vi "Replace Array Element (by ref) [U32].vi"(8 "Error In":errorcluster, 9 "Index":i32, 10 "New Element":u32, 11 "Array in":refnum<vi>) -> (0 "Error Out":errorcluster, 3 "Array out":refnum<vi>)   [LabVIEW 2021, in "Arrays.lvlib"]
uses:
  Arrays.lvlib
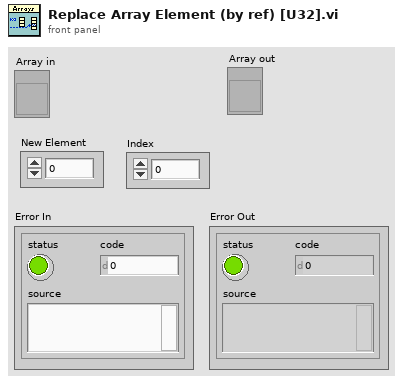
[diagram p1: front panel]
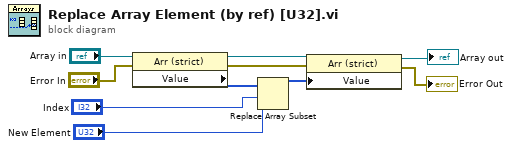
[diagram p0: block diagram]
diagram:
  n1 = property class="Arr (strict)"(reference="Array in", error in="Error In") -> (reference out=w9:refnum<vi>, error out=w5:errorcluster, "Value"=w8:u32[])
  n2 = Replace Array Subset(array=w8, new element="New Element", index="Index") -> (w7:u32[])
  n3 = property class="Arr (strict)"(reference=w9, error in=w5, "Value"=w7) -> (reference out=→"Array out":refnum<vi>, error out=→"Error Out":errorcluster)
